vi "Generate MeasurementLink Server Internal.vi"() -> ()   [LabVIEW 2020]
panel:
  out "error out":errorcluster
  in  "error in (no error)":errorcluster
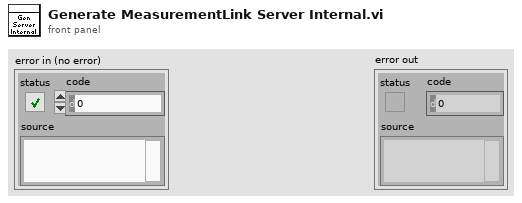
[diagram p1: front panel]
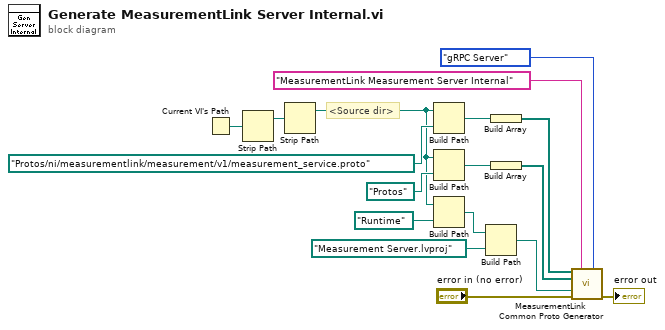
[diagram p0: block diagram]
diagram:
  # "<Source dir>"
  n1 = Current VI's Path() -> (path=w12:path)
  n2 = Strip Path(path=w12) -> (stripped path=w11:path)  [unwired: 1 out]
  n3 = Strip Path(path=w11) -> (stripped path=w13:path)  [unwired: 1 out]
  n4 = Build Path(base path=w13, name or relative path=path "Protos/ni/measurementlink/measurement/v1/measurement_service.proto" ("Proto File Path")) -> (appended path=w16:path)
  n5 = Build Path(base path=w13, name or relative path=path "Protos" ("Proto File Path")) -> (appended path=w14:path)
  n6 = Build Path(base path=w13, name or relative path=path "Runtime" ("Target Project")) -> (appended path=w8:path)
  n7 = Build Path(base path=w8, name or relative path=path "Measurement Server.lvproj" ("Target Project")) -> (appended path=w1:path)
  n8 = Build Array(w16) -> (w3:path[])
  n9 = Build Array(w14) -> (w4:path[])
  n10 = call "MeasurementLink Common Proto Generator.vi"("Proto File Path"=w3, "Generated Library Full Name"="MeasurementLink Measurement Server Internal" ("Generated Library Name"), "Generate"=enum16{"gRPC Server", "gRPC Client", "Both"}."gRPC Server", "Import Paths"=w4, "Target Project"=w1, "error in (no error)"="error in (no error)") -> ("error out"=→"error out":errorcluster)  [unwired: 9 in]
